vi "Get IController .NET.vi"(11 "IController in":refnum<class "IController.lvclass">) -> (2 "IController":refnum<k24>, 3 "IController out":refnum<class "IController.lvclass">)   [LabVIEW 2024, in "SourceGrid.lvlib" / "IController.lvclass"]
uses:
  IController.lvclass
  D:/git/Sourcegrid-LabVIEW/dll/SourceGrid.dll
  dll/SourceGrid.dll
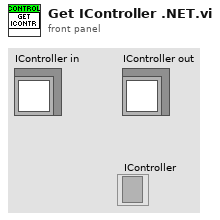
[diagram p1: front panel]
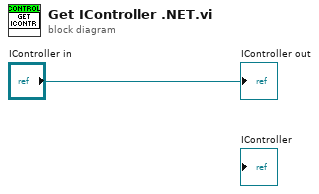
[diagram p0: block diagram]
diagram:
  "IController out" <- "IController in"
